vi "MH_ReadPTUHeader.vi"(8 "entrée d'erreur":errorcluster, 11 "FilePath":path) -> (0 "sortie d'erreur":errorcluster, 1 "TagString":string, 2 "TagArray":T1(array[cluster]) {"TagType" format="%x"}, 3 "refnum Out":refnum<file>, 4 "Cancelled":bool)   [LabVIEW 2019]
panel:
  out "TagTypes":string[](array[string])
  out "n_hdr_items":i32=80
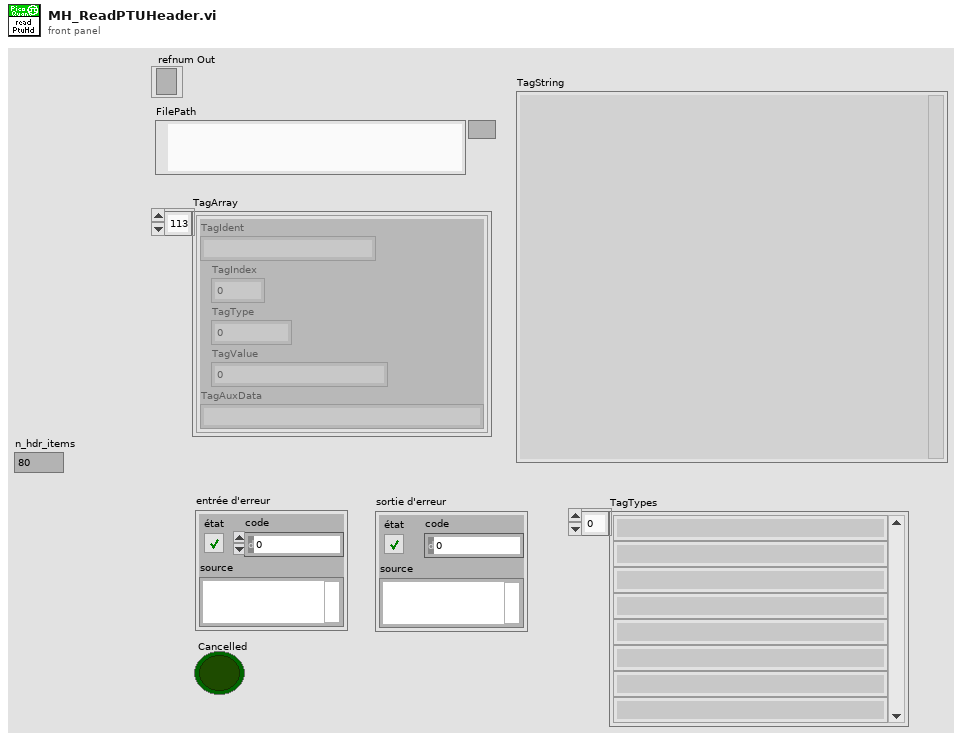
[diagram p1: front panel]
types:
  T1 = cluster{"TagIdent":string, "TagIndex":i32, "TagType":i32, "TagValue":i64, "TagAuxData":string}[]
  T2 = cluster{"TagIdent":string, "TagIndex":i32, "TagType":i32, "TagValue":i64, "TagAuxData":string}
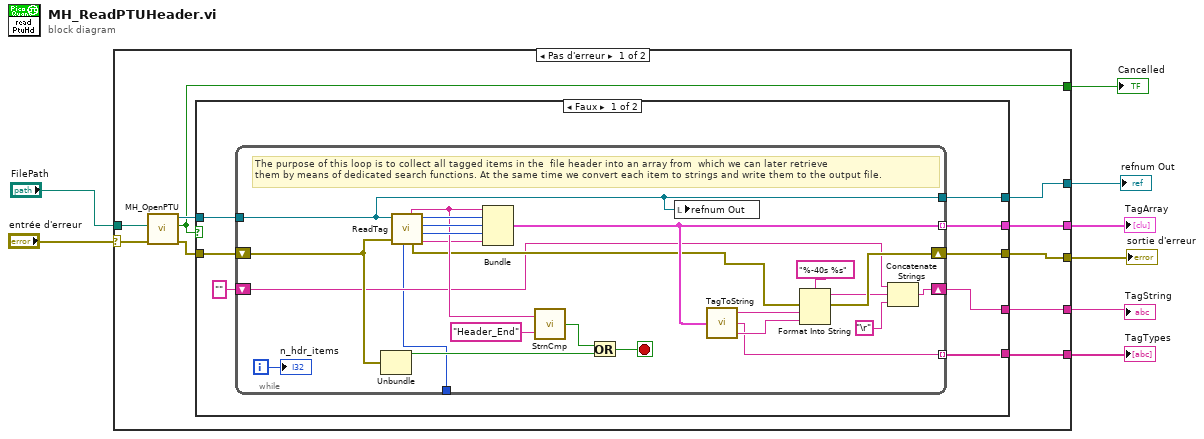
[diagram p0: block diagram]
diagram:
  n1 = case shown="Pas d'erreur" "entrée d'erreur" {
    selector: "entrée d'erreur" -> [w12 w52]
    tunnel: [w18 w52] -> w8
    tunnel: [w17 _] -> w6
    tunnel: [w16 _] -> w5
    tunnel: [w15 _] -> w4
    tunnel: [w11 _] -> w3
    tunnel: "FilePath" -> [w10 _]
    tunnel: [w9 _] -> w1
    frame No Error {
      n2 = call <userlib>:"MH_OpenPTU.vi"("ErrorIn"=w12, "chemin sélectionné"=w10) -> ("ErrorOut"=w13:errorcluster, "Cancelled"=w9:bool, "refnum en sortie"=w14:refnum<file>)  [unwired: 7 in]
      n3 = case shown="Faux" w9 {
        tunnel: w13 -> [w26 w51]
        tunnel: [w25 w51] -> w18
        tunnel: [w24 _] -> w17
        tunnel: [w23 _] -> w16
        tunnel: [w22 _] -> w15
        tunnel: w14 -> [w21 _]
        tunnel: [w19 _] -> w11
        frame False {
          n4 = while {
            shift-left: w26 -> [w49]
            shift-right: [w37] -> w25
            tunnel: w21 -> [w27]
            tunnel: [w39] -> w22 mode=indexing
            tunnel: [w27] -> w23
            shift-right: [w31] -> w24
            shift-left: "" -> [w30]
            tunnel: [w29] -> w19 mode=indexing
            tunnel: [w28] -> _
            i -> [w45]
            stop <- w50 stop-if-true
            # "The purpose of this loop is to collect all tagged items in the  file header into an array from  which we can later retrieve \nthem by means of dedicated search functions. At the same time we convert each item to strings and write them to the output file."
            n5 = Unbundle(w49) -> ("status"=w42:bool)  [unwired: 2 out]
            n6 = call <userlib>:"ReadTag.vi"("refnum"=w27, "error in"=w49) -> ("offset (en octets)"=w28:i64, "TagIdent"=w41:string, "TagIndex"=w48:i32, "TagType"=w47:i32, "error out"=w33:errorcluster, "TagValue"=w46:i64, "TagAuxData"=w40:string)  [unwired: 2 in]
            n7 = Bundle("TagIdent"=w41, "TagIndex"=w48, "TagType"=w47, "TagValue"=w46, "TagAuxData"=w40) -> (w39:T2)  [unwired: 1 in]
            n8 = call <userlib>:"StrnCmp.vi"("String 2"="Header_End", "String 1"=w41) -> ("equal"=w43:bool)
            n9 = Or(x=w43, y=w42) -> (x .or. y?=w50:bool)
            n10 = local write "refnum Out"(w27) -> ()
            n11 = call <userlib>:"TagToString.vi"("TagData"=w39) -> ("StrTagValue"=w35:string, "StrTagType"=w29:string, "StrTagName"=w34:string)  [unwired: 2 in]
            n12 = Format Into String(format string="%-40s %s", error in=w33, w34, w35) -> (resulting string=w36:string, error out=w37:errorcluster)  [unwired: 1 in]
            n13 = Concatenate Strings(w30, w36, "\r") -> (w31:string)
            "n_hdr_items" <- w45
          }
        }
        frame True {
        }
      }
    }
    frame Error {
    }
  }
  "sortie d'erreur" <- w8
  "TagString" <- w6
  "refnum Out" <- w5
  "TagArray" <- w4
  "TagTypes" <- w3
  "Cancelled" <- w1
